vi "Configure Trigger (Runt).vi"(0 "VISA resource name":refnum<visa-resource-name>, 1 "Enable Time Qualified Runt Pulse (F: Disable)":bool, 5 "Trigger Source (1: Channel1)":i32(ring)=1 items=["Channel1"=1, "Channel2"=2, "Channel3"=3, "Channel4"=4], 9 "Trigger Polarity (0: Negative)":i32(ring) items=["Negative", "Positive"], 11 "error in (no error)":errorcluster, 12 "Runt Time (1E-9 s)":dbl=1e-09) -> (4 "VISA resource name out":refnum<visa-resource-name>, 15 "error out":errorcluster)   [LabVIEW 2020, in "Agilent 90000 Series.lvlib"]
doc: "Configures runt trigger parameters."
uses:
  Agilent 90000 Series.lvlib
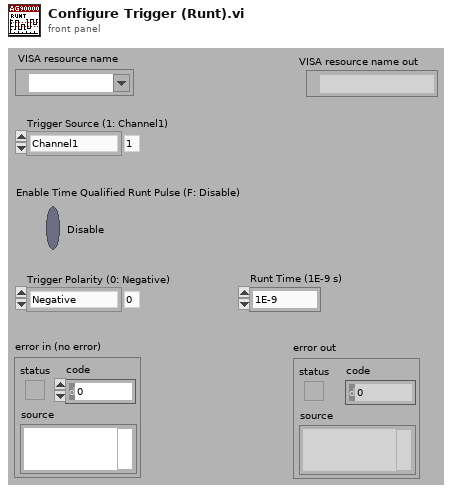
[diagram p1: front panel]
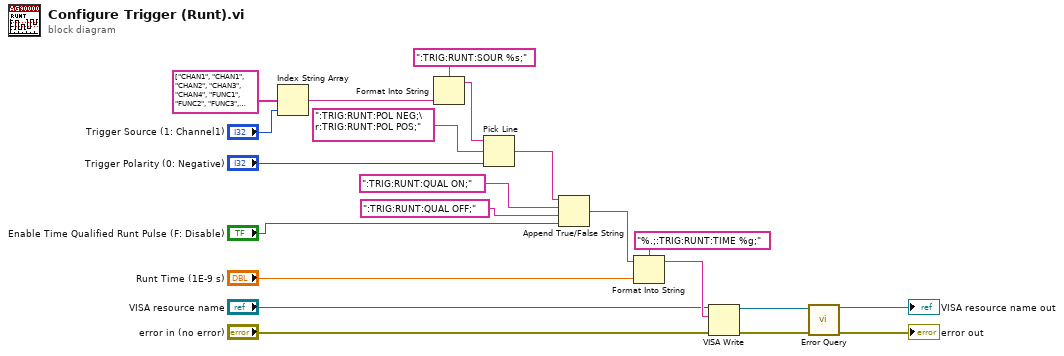
[diagram p0: block diagram]
diagram:
  n1 = Index String Array(1:"Trigger Source (1: Channel1)", 2:string[] ["CHAN1", "CHAN1", "CHAN2", "CHAN3", "CHAN4", "FUNC1", "FUNC2", "FUNC3", "FUNC4", "WMEM1", "WMEM2", "WMEM3", "WMEM4", "AUX", "LINE"]) -> (0:w1:string)  [unwired: 1 out]
  n2 = Format Into String(format string=":TRIG:RUNT:SOUR %s;", w1) -> (resulting string=w2:string)  [unwired: 2 in, 1 out]
  n3 = Pick Line(string ("")=w2, multi-line string=":TRIG:RUNT:POL NEG;\r:TRIG:RUNT:POL POS;", line index="Trigger Polarity (0: Negative)") -> (output string=w19:string)
  n4 = Append True/False String(1:"Enable Time Qualified Runt Pulse (F: Disable)", 2:":TRIG:RUNT:QUAL OFF;", 3:":TRIG:RUNT:QUAL ON;", 4:w19) -> (0:w15:string)
  n5 = Format Into String(format string="%.;:TRIG:RUNT:TIME %g;", initial string=w15, "Runt Time (1E-9 s)") -> (resulting string=w12:string)  [unwired: 1 in, 1 out]
  n6 = VISA Write(VISA resource name="VISA resource name", write buffer=w12, error in (no error)="error in (no error)") -> (VISA resource name out=w9:refnum<visa-resource-name>, error out=w8:errorcluster)  [unwired: 1 out]
  n7 = call "Error Query.vi"("error in (no error)"=w8, "VISA resource name"=w9) -> ("error out"=→"error out":errorcluster, "VISA resource name out"=→"VISA resource name out":refnum<visa-resource-name>)  [unwired: 8 out]
